vi "editscenario handle preview.vi"(6 "user":string, 8 "error in (no error)":errorcluster, 10 "sxScenarioId (\"\")":string, 11 "Connection Refnum":T1) -> (0 "error out":errorcluster, 2 "image":string, 3 "dup Connection Refnum":T1)   [LabVIEW 2011]
uses:
  SI.LIB/ODBC/SQL Controls/Connection Refnum.ctl
  server/DIAdem/Datasheet/Datasheet Generator Settings.ctl
panel:
  in  "nopreview.png":string
  in  "error.png":string
  in  "missing.png":string
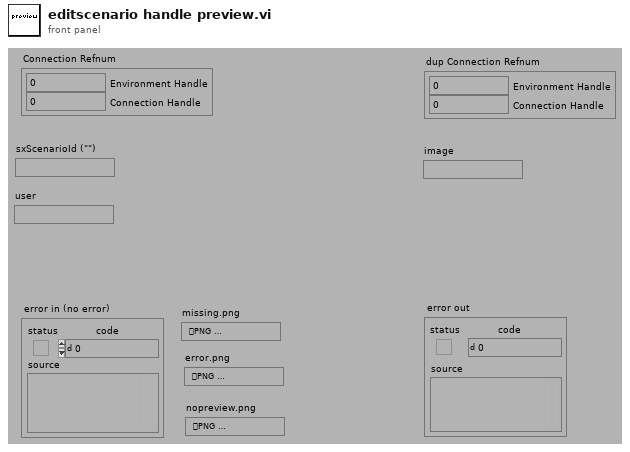
[diagram p1: front panel]
types:
  T1 = typedef "Connection Refnum.ctl" = cluster{"Environment Handle":i32, "Connection Handle":i32}
  T2 = typedef "Template Record.ctl" = cluster{"ixTemplate":i32, "sxTemplateId":string, "sDescription":string, "sCreator":string, "tCreationDate":timestamp, "sModifier":string, "tModifiedDate":timestamp, "sType":string, "sStyle":string, "sFormat":string, "dWidth":dbl, "dHeight":dbl, "sFilename":string, "sScript":string, "sLayout":string, "sEditor":string, "sStyleProcess":string}
  T3 = typedef "DATASHEET Generator Settings.ctl" = cluster{"Wait? (t)":bool, "ClientPrint? (f)":bool, "Client (\"\")":string, "joinPDF":bool, "Sort Method":enum16{"Item", "Template", "No Sort"}, "Export Row (-1=all)":i32, "Preview":bool, "Estimate Time":bool, "username":string, "jobid":string}
  T4 = typedef "Datasheet Report Info.ctl" = cluster{"sxTemplateId":string[], "reportPath":path}
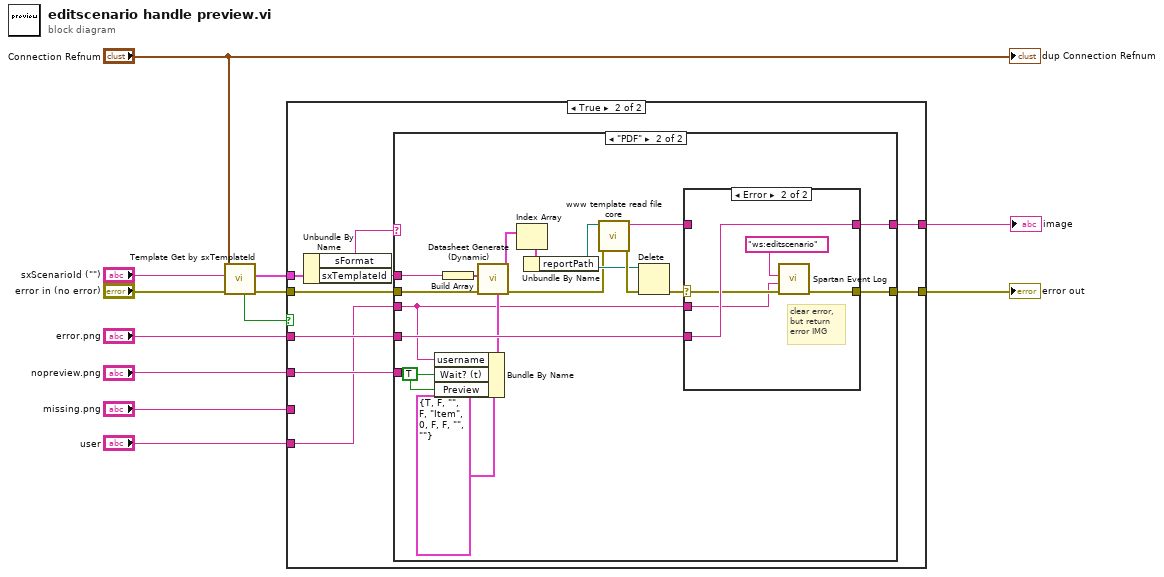
[diagram p0: block diagram]
diagram:
  n1 = call "Template Get by sxTemplateId.vi"("error in (no error)"="error in (no error)", "sxTemplateId (\"\")"="sxScenarioId (\"\")", "Connection Refnum"="Connection Refnum") -> ("error out"=w1:errorcluster, "Template Record"=w9:T2, "Data Present"=w7:bool)  [unwired: 6 out]
  n2 = case shown="True" w7 {
    tunnel: w9 -> [_ w23]
    tunnel: [w13 w20] -> w2
    tunnel: [w14 w21] -> w8
    tunnel: "error.png" -> [_ w18]
    tunnel: "missing.png" -> [w14 _]
    tunnel: "nopreview.png" -> [_ w17]
    tunnel: "user" -> [_ w16]
    tunnel: w1 -> [w13 w15]
    frame False {
    }
    frame True {
      n3 = Unbundle By Name(w23) -> ("sFormat"=w19:string, "sxTemplateId"=w22:string)
      n4 = case shown="\"PDF\"" w19 {
        tunnel: w22 -> [_ w42]
        tunnel: [w25 w38] -> w21
        tunnel: [w24 w37] -> w20
        tunnel: w18 -> [_ w36]
        tunnel: w17 -> [w25 _]
        tunnel: w16 -> [_ w28]
        tunnel: w15 -> [w24 w27]
        frame "no Preview", Default {
        }
        frame "PDF" {
          w32 = TRUE ("Wait? (t)")
          n5 = Bundle By Name(cluster=T3 {"Wait? (t)"=TRUE, "ClientPrint? (f)"=FALSE, "Client (\"\")"="", "joinPDF"=FALSE, "Sort Method"=enum."Item", "Export Row (-1=all)"=0, "Preview"=FALSE, "Estimate Time"=FALSE, "username"="", "jobid"=""} ("Generator Settings"), "username"=w28, "Wait? (t)"=w32, "Preview"=w32) -> (w30:T3)
          n6 = Build Array(w42) -> (w33:string[])
          n7 = call "Datasheet Generate (Dynamic).vi"("Generator Settings"=w30, "error in (no error)"=w27, "Templates"=w33) -> ("error out"=w26:errorcluster, "Datasheet Paths"=w35:T4[])  [unwired: 6 in, 1 out]
          n8 = Index Array(array=w35) -> (element=w34:T4)  [unwired: 1 in]
          n9 = Unbundle By Name(w34) -> ("reportPath"=w29:path)
          n10 = call "www template read file core.vi"("error in (no error)"=w26, "Path"=w29) -> ("error out"=w41:errorcluster, "File Content"=w39:string)  [unwired: 8 out]
          n11 = Delete(path (use dialog)=w29, error in=w41) -> (error out=w40:errorcluster)  [unwired: 5 out]
          n12 = case shown="Error" w40 {
            selector: w40 -> [w43 w48]
            tunnel: w39 -> [w44 _]
            tunnel: [w44 w49] -> w38
            tunnel: [w43 w47] -> w37
            tunnel: w36 -> [_ w49]
            tunnel: w28 -> [_ w46]
            frame No Error {
            }
            frame Error {
              # "clear error,\nbut return\nerror IMG"
              n13 = call "Spartan Event Log.vi"("error in (no error)"=w48, "username (\"\")"=w46, "module (\"\")"="ws:editscenario" ("user")) -> ("error out"=w47:errorcluster)  [unwired: 5 in]
            }
          }
        }
      }
    }
  }
  "error out" <- w2
  "image" <- w8
  "dup Connection Refnum" <- "Connection Refnum"
